vi "tagDB TagsChanged.vi"(8 "error in (no error)":errorcluster, 11 "DB Ref":T1) -> (0 "error in (no error) (dup)":errorcluster, 2 "item changed?":bool, 3 "DB Ref (dup)":T1)   [LabVIEW 2014, in "TagDB(dev).lvlib"]
doc: "[Covers: REQ_API_DBITEMCHANGED]"
uses:
  TagDB(dev).lvlib
  tagDB_Def.ctl
  Private/_Cast TagDB Ref to DVR.vi
  Error/_[error50000]Invalid DB REF.vi
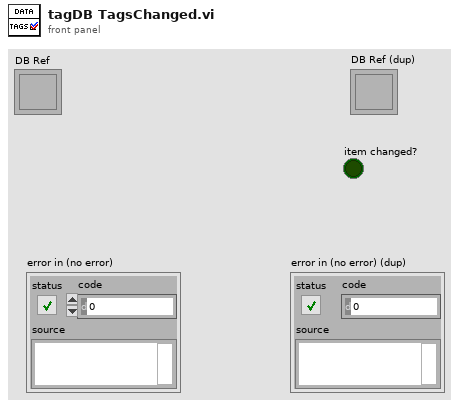
[diagram p1: front panel]
types:
  T1 = typedef "TagDB(dev).lvlib/tagDB_Def.ctl" = refnum<k1>
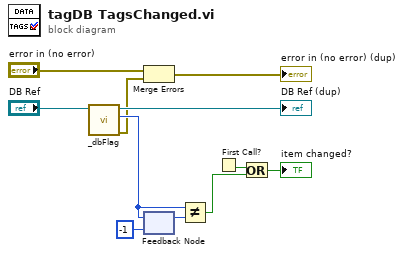
[diagram p0: block diagram]
diagram:
  n1 = call "_dbFlag.vi"("DB Ref"="DB Ref") -> ("error in (no error) (dup)"=w2:errorcluster, "DataItemFlag"=w4:i64, "DB Ref (dup)"=→"DB Ref (dup)":T1)  [unwired: 8 in]
  n2 = Merge Errors("error in (no error)", w2) -> (→"error in (no error) (dup)":errorcluster)
  n3 = feedback-in #1(w4) -> ()
  n4 = feedback #1(i64 -1 ("DataItemFlag")) -> (w10:i64)
  n5 = Not Equal?(x=w4, y=w10) -> (x != y?=w9:bool)
  n6 = First Call?() -> (First Call?: T/F=w8:bool)
  n7 = Or(x=w8, y=w9) -> (x .or. y?=→"item changed?":bool)
